vi "SSH_WriteLines.vi"(8 "error in (no error)":errorcluster, 10 "Send":string, 11 "Python in":cluster{"Python":refnum<k35>, "py file":path}) -> (0 "error out":errorcluster, 1 "Rest":string, 2 "Reply":string, 3 "Python out":cluster{"Python":refnum<k35>, "py file":path})   [LabVIEW 2020]
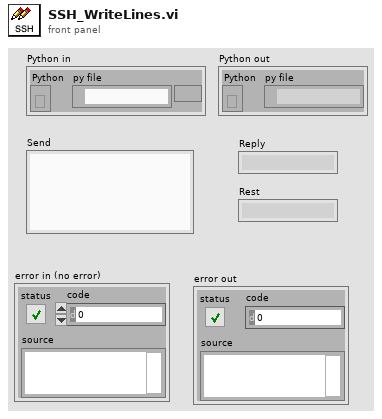
[diagram p1: front panel]
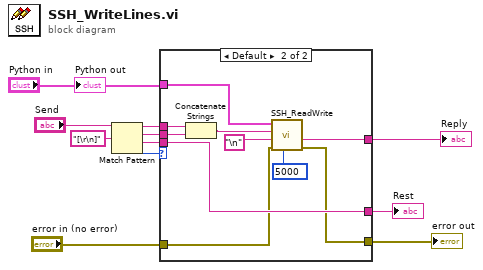
[diagram p0: block diagram]
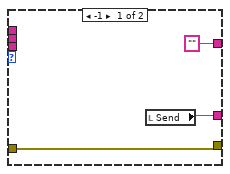
[diagram p2: hidden frame]
diagram:
  n1 = Match Pattern(string="Send", regular expression="[\r\n]") -> (before substring=w11:string, match substring=w9:string, after substring=w4:string, offset past match=w6:i32)  [unwired: 1 in]
  n2 = case shown="Default" w6 {
    tunnel: w11 -> [_ w24]
    tunnel: w9 -> [_ w21]
    tunnel: "Python in" -> [_ w19]
    tunnel: ["" ("Console") w18] -> w8
    tunnel: [w13 w17] -> w5
    tunnel: w4 -> [_ w17]
    tunnel: "error in (no error)" -> [w12 w16]
    tunnel: [w12 w15] -> w1
    frame -1 {
      n3 = local read "Send"() -> (w13:string)
    }
    frame Default {
      n4 = Concatenate Strings(w24, w21) -> (w22:string)
      n5 = call "SSH_ReadWrite.vi"("Timeout (ms)"=u32 5000, "error in (no error)"=w16, "Wait for"="\n" ("search string"), "To Send"=w22, "Python in"=w19) -> ("error out"=w15:errorcluster, "Console"=w18:string)  [unwired: 5 in]
    }
  }
  "Reply" <- w8
  "Rest" <- w5
  "error out" <- w1
  "Python out" <- "Python in"
